vi "Set Variable.vi"(8 "error in (no error)":errorcluster, 9 "Value":variant, 10 "Name":string, 11 "Execution in":refnum<data-value>) -> (0 "error out":errorcluster, 3 "Execution out":refnum<data-value>)   [LabVIEW 2015, in "Execution.lvclass"]
uses:
  Execution.lvclass
  Project.lvclass
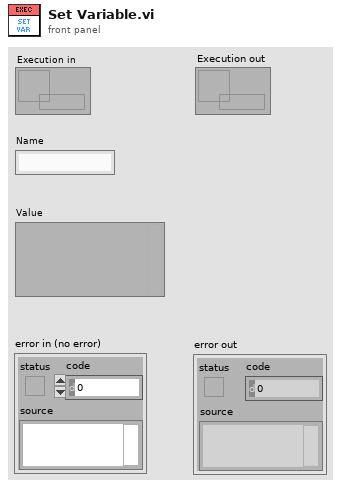
[diagram p1: front panel]
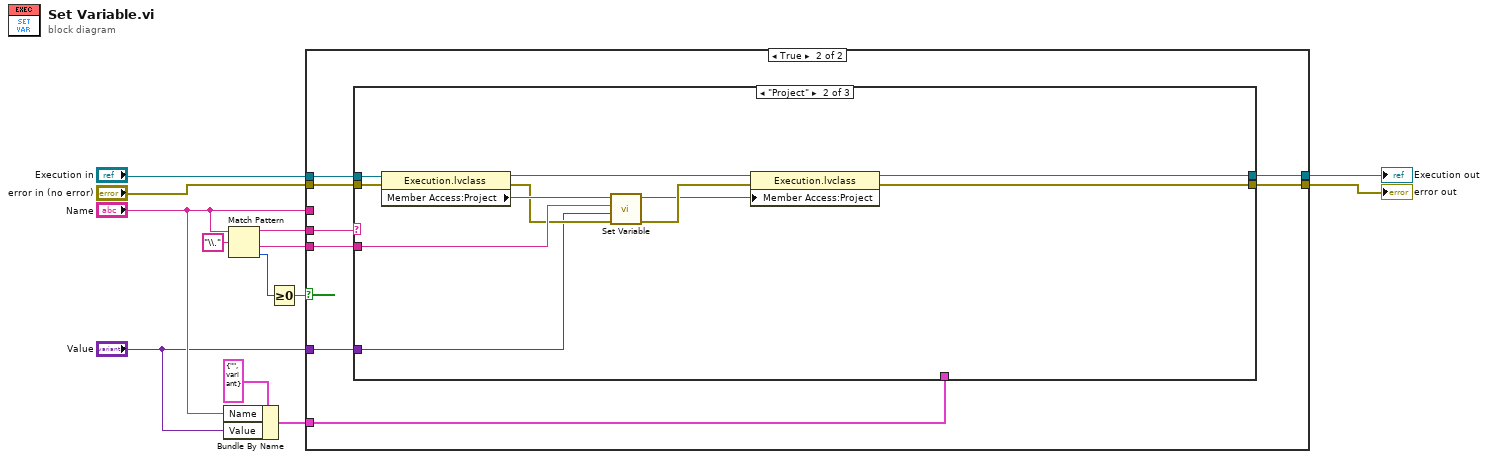
[diagram p0: block diagram]
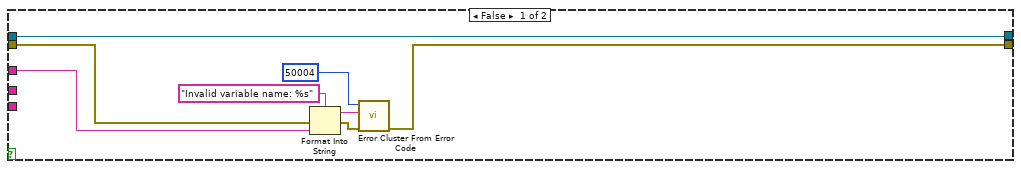
[diagram p2: hidden frame]
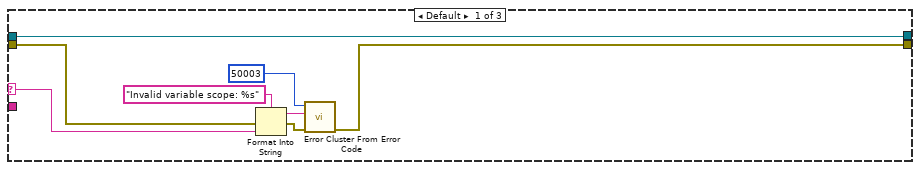
[diagram p3: hidden frame]
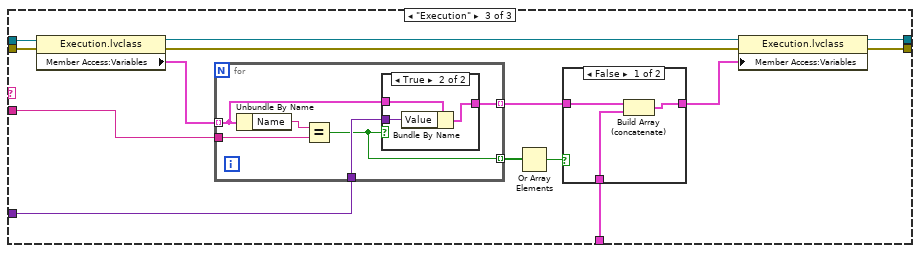
[diagram p4: hidden frame]
diagram:
  n1 = Bundle By Name(cluster=cluster{"Name":string, "Value":variant} {"Name"="", "Value"=variant} ("Variable"), "Name"="Name", "Value"="Value") -> (w2:cluster{"Name":string, "Value":variant})
  n2 = Match Pattern(string="Name", regular expression="\\.") -> (before substring=w9:string, after substring=w10:string, offset past match=w12:i32)  [unwired: 1 in, 1 out]
  n3 = Greater Or Equal To 0?(x=w12) -> (x >= 0?=w11:bool)
  n4 = case shown="True" w11 {
    tunnel: w10 -> [_ w27]
    tunnel: w9 -> [_ w29]
    tunnel: "Execution in" -> [w17 w28]
    tunnel: "error in (no error)" -> [w16 w26]
    tunnel: [w17 w25] -> w6
    tunnel: [w14 w24] -> w1
    tunnel: "Name" -> [w15 _]
    tunnel: "Value" -> [_ w23]
    tunnel: w2 -> [_ w22]
    frame False {
      n5 = Format Into String(format string="Invalid variable name: %s" ("error message (\"\")"), error in=w16, w15) -> (resulting string=w20:string, error out=w19:errorcluster)  [unwired: 1 in]
      n6 = call <vilib>:"Error Cluster From Error Code.vi"("error in (no error)"=w19, "error message (\"\")"=w20, "error code (0)"=50004) -> ("error out"=w14:errorcluster)  [unwired: 6 in]
    }
    frame True {
      n7 = case shown="\"Project\"" w29 {
        selector: w29 -> [w31 _ _]
        tunnel: w28 -> [w37 w48 w62]
        tunnel: w27 -> [_ w46 w60]
        tunnel: w26 -> [w32 w45 w61]
        tunnel: [w37 w40 w51] -> w25
        tunnel: [w30 w39 w50] -> w24
        tunnel: w23 -> [_ w43 w58]
        tunnel: w22 -> [_ _ w54]
        frame Default {
          n8 = Format Into String(format string="Invalid variable scope: %s" ("error message (\"\")"), error in=w32, w31) -> (resulting string=w35:string, error out=w34:errorcluster)  [unwired: 1 in]
          n9 = call <vilib>:"Error Cluster From Error Code.vi"("error in (no error)"=w34, "error message (\"\")"=w35, "error code (0)"=50003) -> ("error out"=w30:errorcluster)  [unwired: 6 in]
        }
        frame "Project" {
          n10 = property class="Execution.lvclass"(reference=w48, error in=w45) -> (reference out=w42:refnum<data-value>, error out=w44:errorcluster, "Member Access:Project"=w47:refnum<class "Project.lvclass">)
          n11 = call-dynamic "Set Variable.vi"("error in (no error)"=w44, "Value"=w43, "Name"=w46, "Project in"=w47) -> ("error out"=w41:errorcluster, "Project out"=w38:refnum<class "Project.lvclass">)  [unwired: 6 in]
          n12 = property class="Execution.lvclass"(reference=w42, error in=w41, "Member Access:Project"=w38) -> (reference out=w40:refnum<data-value>, error out=w39:errorcluster)
        }
        frame "Execution" {
          n13 = property class="Execution.lvclass"(reference=w62, error in=w61) -> (reference out=w53:refnum<data-value>, error out=w52:errorcluster, "Member Access:Variables"=w59:cluster{"Name":string, "Value":variant}[])
          n14 = for {
            tunnel: w60 -> [w71]
            tunnel: w59 -> [w70] mode=indexing
            tunnel: w58 -> [w69]
            tunnel: [w68] -> w55 mode=indexing
            tunnel: [w67] -> w57 mode=indexing
            n15 = Unbundle By Name(w70) -> ("Name"=w72:string)
            n16 = Equal?(x=w72, y=w71) -> (x = y?=w67:bool)
            n17 = case shown="True" w67 {
              tunnel: w70 -> [w73 w76]
              tunnel: w69 -> [_ w75]
              tunnel: [w73 w74] -> w68
              frame False {
              }
              frame True {
                n18 = Bundle By Name(cluster=w76, "Value"=w75) -> (w74:cluster{"Name":string, "Value":variant})
              }
            }
          }
          n19 = Or Array Elements(Boolean array=w57) -> (logical OR=w56:bool)
          n20 = case shown="False" w56 {
            tunnel: w55 -> [w65 w66]
            tunnel: w54 -> [w64 _]
            tunnel: [w63 w66] -> w49
            frame False {
              n21 = Build Array (concatenate)(w65, w64) -> (w63:cluster{"Name":string, "Value":variant}[])
            }
            frame True {
            }
          }
          n22 = property class="Execution.lvclass"(reference=w53, error in=w52, "Member Access:Variables"=w49) -> (reference out=w51:refnum<data-value>, error out=w50:errorcluster)
        }
      }
    }
  }
  "error out" <- w1
  "Execution out" <- w6
